vi "NIFPGA-MCS.close.vi"(0 "i ref in":refnum<vi>, 3 "ms timeout (10000)":i32=10000, 5 "error in (no error)":errorcluster) -> (14 "i ref out":refnum<vi>, 17 "timed out":bool, 19 "error out":errorcluster)   [LabVIEW 2014, in "NIFPGA-MCS.lvlib"]
doc: "Closes the connection to the MCS."
uses:
  NIFPGA-MCS.lvlib
  CSinstr.lib/NI-FPGA-MCS/host/instrumentDriver/fpga_vi_ref.ctl
  CSCore/CSApplicationBaseClasses/DeviceBase/DeviceBase.lvlib
  CSinstr.lib/NI-FPGA-MCS/host/instrumentDriver/NI-FPGA-MCS_Driver.lvlib
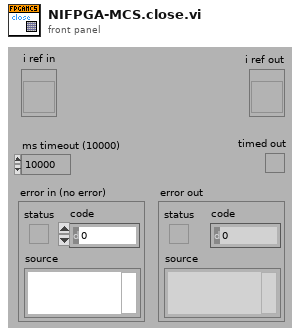
[diagram p1: front panel]
types:
  T1 = typedef "NIFPGA-MCS.lvlib/NIFPGA-MCS.i attribute.ctl" = cluster{"fpgaViRef":T2}
  T2 = typedef "NI-FPGA-MCS_Driver.lvlib/fpga_vi_ref.ctl" = refnum<k20>
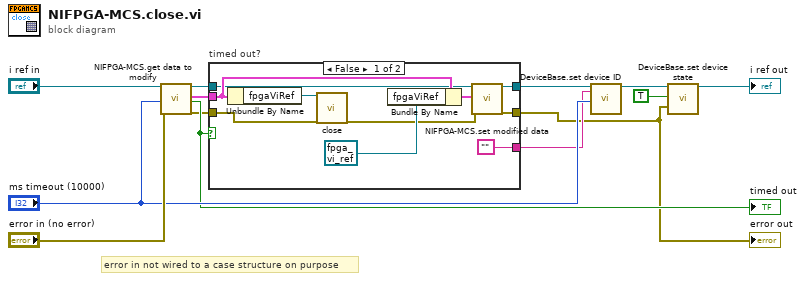
[diagram p0: block diagram]
diagram:
  # "error in not wired to a case structure on purpose"
  n1 = call "NIFPGA-MCS.get data to modify.vi"("i ref in"="i ref in", "ms timeout (10000)"="ms timeout (10000)", "error in (no error)"="error in (no error)") -> ("i ref out"=w8:refnum<vi>, "i attribute"=w6:T1, "timed out"=w9:bool, "error out"=w7:errorcluster)  [unwired: 13 in]
  "timed out" <- w9
  n2 = case "timed out?" shown="False" w9 {
    tunnel: w8 -> [w15 w25]
    tunnel: w7 -> [w23 w24]
    tunnel: w6 -> [w19 _]
    tunnel: [w21 w25] -> w5
    tunnel: [w20 w24] -> w1
    tunnel: ["" _] -> w2
    frame False {
      n3 = Unbundle By Name(w19) -> ("fpgaViRef"=w18:T2)
      n4 = call "close.vi"("fpga_vi_ref"=w18, "error in (no error)"=w23) -> ("error out"=w16:errorcluster)  [unwired: 17 in]
      n5 = Bundle By Name(cluster=w19, "fpgaViRef"=T2 refnum) -> (w22:T1)
      n6 = call "NIFPGA-MCS.set modified data.vi"("i ref in"=w15, "i attribute"=w22, "error in (no error)"=w16) -> ("i ref out"=w21:refnum<vi>, "error out"=w20:errorcluster)  [unwired: 15 in]
    }
    frame True {
    }
  }
  "error out" <- w1
  n7 = call "DeviceBase.set device ID.vi"("i ref in"=w5, "deviceID"=w2, "ms timeout (10000)"="ms timeout (10000)") -> ("i ref out"=w4:refnum<vi>)  [unwired: 14 in, 2 out]
  n8 = call "DeviceBase.set device state.vi"("i ref in"=w4, "implicit"=TRUE, "device error"=w1) -> ("i ref out"=→"i ref out":refnum<vi>)  [unwired: 14 in, 2 out]
